vi "SPI Write.vi"(5 "buffer":string, 6 "options":u32=6 format="%02x", 8 "error in (no error)":errorcluster, 9 "Bytes To Send":u32, 11 "handle":u32 format="%08x") -> (0 "error out":errorcluster, 2 "sizeTransfered":u32, 3 "handle out":u32 format="%08x")   [LabVIEW 2018, in "libMPSSE-SPI.lvlib"]
doc: "FTDI_API FT_STATUS SPI_Write(FT_HANDLE handle, uint8 *buffer,\n uint32 sizeToTransfer, uint32 *sizeTransfered, uint32 options);"
uses:
  libMPSSE-SPI.lvlib
  dll/libMPSSE.dll
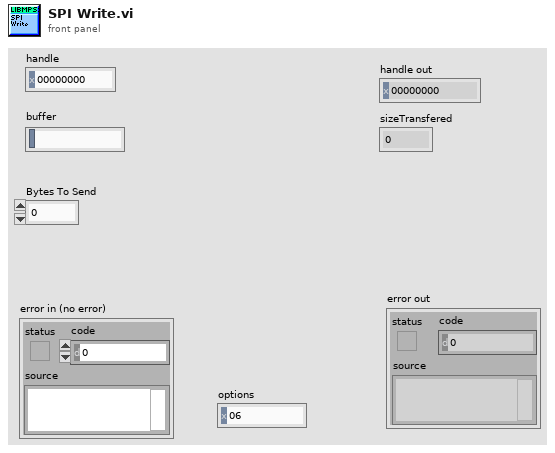
[diagram p1: front panel]
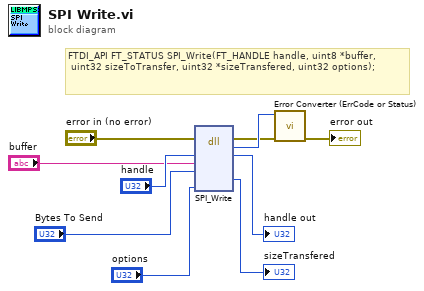
[diagram p0: block diagram]
diagram:
  # "FTDI_API FT_STATUS SPI_Write(FT_HANDLE handle, uint8 *buffer,\n\tuint32 sizeToTransfer, uint32 *sizeTransfered, uint32 options);"
  n1 = dll-call lib="D:/LABVIEW/SEQUENSER SNA/Ver 03/FTDI SPI/dll/libMPSSE.*" fn="SPI_Write"(error in="error in (no error)", "handle"="handle", "buffer"="buffer", "sizeToTransfer"="Bytes To Send", "options"="options") -> (error out=w4:errorcluster, "return type"=w10:u32, "handle"=→"handle out":u32, "sizeTransfered"=→"sizeTransfered":u32)  [unwired: 6 in, 1 out]
  n2 = call "Error Converter (ErrCode or Status).vi"("error in (no error)"=w4, "error code"=w10) -> ("error out"=→"error out":errorcluster)  [unwired: 9 in]
